vi "set_gate_parameters.vi"(4 "repetitions":i64, 5 "pulse duration (iterations)":i64, 6 "offset duration (iterations)":i64, 7 "clock index":i32, 8 "error in (no error)":errorcluster, 9 "low phase duration (iterations)":i64, 10 "high phase duration (iterations)":i64, 11 "FPGAWrapperAN110607Galvo in":refnum<class "FPGAWrapperAN110607Galvo.lvclass">) -> (0 "error out":errorcluster, 3 "FPGAWrapperAN110607Galvo out":refnum<class "FPGAWrapperAN110607Galvo.lvclass">)   [LabVIEW 2010, in "FPGAWrapperAN110607Galvo.lvclass"]
uses:
  FPGAWrapperAN110607Galvo.lvclass
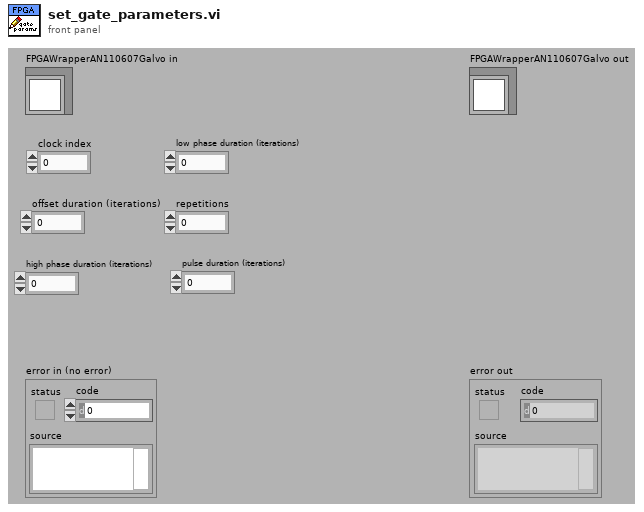
[diagram p1: front panel]
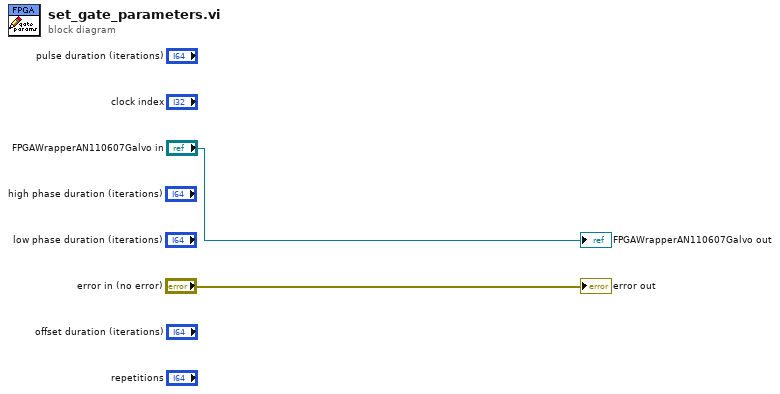
[diagram p0: block diagram]
diagram:
  "error out" <- "error in (no error)"
  "FPGAWrapperAN110607Galvo out" <- "FPGAWrapperAN110607Galvo in"
